vi "Add overlay to merged image.vi"(2 "Image in":T1, 3 "File paths":path[](array[path]), 4 "error in":errorcluster, 5 "Overlay frame numbers":u32[](array[numeric]), 6 "Black/White levels":cluster{ext, ext}[](array[cluster]), 7 "Overlay colors":u32[](array[numeric])) -> (0 "error out":errorcluster, 1 "Image Out":T1)   [LabVIEW 2011]
doc: "Writes the text overlay on the merged images."
uses:
  <vilib>/vision/Image Controls.llb/IMAQ Image.ctl
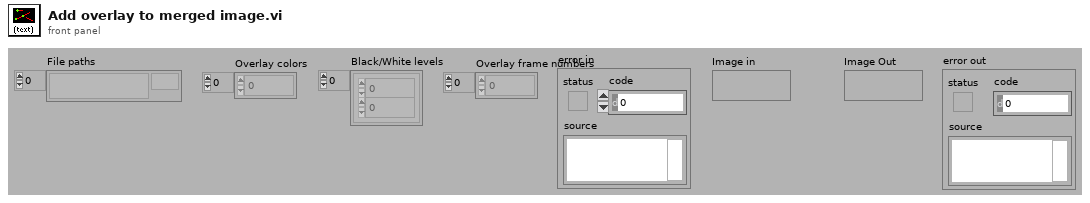
[diagram p1: front panel]
types:
  T1 = typedef "IMAQ Image.ctl" = refnum<image>
  T2 = cluster{"Desired Font (Application)":enum16{"User-specified Font", "Application Font", "System Font", "Dialog Font"}, "[User-specified Font]":cluster{"Font Name":string, "Size":i16, "Strikeout?":bool, "Italic?":bool, "Underline?":bool, "Outline?":bool, "Shadow?":bool, "Bold?":bool, "Rotation Angle":dbl}, "Horizontal Alignment":i16, "Vertical Alignment":i16}
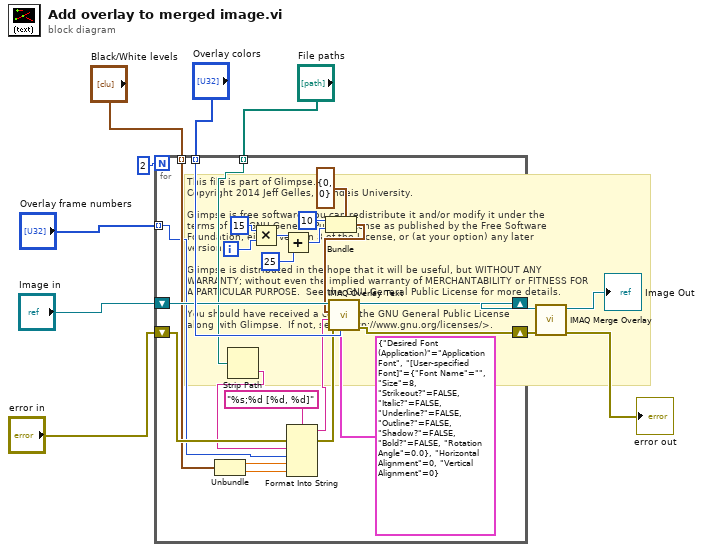
[diagram p0: block diagram]
diagram:
  # "This file is part of Glimpse. \nCopyright 2014 Jeff Gelles, Brandeis University.    \n\nGlimpse is free software: you can redistribute it and/or modify it under the \nterms of the GNU General Public License as published by the Free Software \nFoundation, either version 3 of the License, or (at your option) any later \nversion.\n\nGlimpse is distributed in the hope that it will be useful, but WITHOUT ANY \nWARRANTY; without even the implied warranty of MERCHANTABILITY or FITNESS FOR \nA PARTICULAR PURPOSE.  See the GNU General Public License for more details.\n\nYou should have received a copy of the GNU General Public License\nalong with Glimpse.  If not, see <http://www.gnu.org/licenses/>."
  n1 = for {
    N: 2 -> [_]
    tunnel: "Overlay colors" -> [w34] mode=indexing
    shift-right: [w33] -> w7
    shift-left: "error in" -> [w19]
    shift-right: [w31] -> w9
    shift-left: "Image in" -> [w32]
    tunnel: "File paths" -> [w13] mode=indexing
    tunnel: "Black/White levels" -> [w18] mode=indexing
    tunnel: "Overlay frame numbers" -> [w17] mode=indexing
    i -> [w23]
    n2 = Unbundle(w18) -> (w16:ext, w15:ext)
    n3 = Strip Path(path=w13) -> (name=w12:string)  [unwired: 1 out]
    n4 = Multiply(x=15 ("X"), y=w23) -> (x*y=w25:i32)
    n5 = Add(x=w25, y=25 ("X")) -> (x+y=w26:i32)
    n6 = Format Into String(format string="%s;%d [%d, %d]", error in=w19, w12, w17, w16, w15) -> (resulting string=w21:string, error out=w20:errorcluster)  [unwired: 1 in]
    n7 = Bundle(cluster=cluster{"X":i32, "Y":i32} {"X"=0, "Y"=0} ("Origin"), "X"=10, "Y"=w26) -> (w29:cluster{"X":i32, "Y":i32})
    n8 = call "IMAQ Overlay Text"("Text Color (black)"=w34, "Font, Size & Style"=T2 {"Desired Font (Application)"=enum."Application Font", "[User-specified Font]"={"Font Name"="", "Size"=8, "Strikeout?"=FALSE, "Italic?"=FALSE, "Underline?"=FALSE, "Outline?"=FALSE, "Shadow?"=FALSE, "Bold?"=FALSE, "Rotation Angle"=0.0}, "Horizontal Alignment"=0, "Vertical Alignment"=0}, "error in (no error)"=w20, "String"=w21, "Origin"=w29, "Image"=w32) -> ("error out"=w33:errorcluster, "Image Out"=w31:T1)  [unwired: 2 in, 2 out]
  }
  n9 = call "IMAQ Merge Overlay"("error in (no error)"=w7, "Image Src"=w9) -> ("error out"=→"error out":errorcluster, "Image Dst Out"=→"Image Out":T1)  [unwired: 3 in, 5 out]
